vi "RIO control block_Dev_1.0.vi"() -> ()   [LabVIEW 2013]
uses:
  <vilib>/NI/Current Value Table/Type Defs/File Format.ctl
  <vilib>/NI/Current Value Table/Type Defs/Single Tag.ctl
  <vilib>/NI/Current Value Table/Type Defs/Data Types.ctl
  <vilib>/NI/Current Value Table/Type Defs/Tag Grouping set.ctl
  <vilib>/NI/Current Value Table/Type Defs/Group Data.ctl
  <vilib>/NI/Current Value Table/Read tags into grouped data.vi
  <vilib>/NI/Current Value Table/Write grouped data to tags.vi
  <vilib>/NI/Current Value Table/Read Index Set.vi
  <vilib>/NI/Current Value Table/DataTypes/Double_Read Index Set.vi
  <vilib>/NI/Current Value Table/DataTypes/Array of String_Read Index Set.vi
  <vilib>/NI/Current Value Table/DataTypes/Array of Boolean_Read Index Set.vi
  <vilib>/NI/Current Value Table/DataTypes/Array of Single_Read Index Set.vi
  <vilib>/NI/Current Value Table/DataTypes/Array of Double_Read Index Set.vi
  <vilib>/NI/Current Value Table/DataTypes/Array of I8_Read Index Set.vi
  <vilib>/NI/Current Value Table/DataTypes/Array of I16_Read Index Set.vi
  <vilib>/NI/Current Value Table/DataTypes/Array of I32_Read Index Set.vi
  <vilib>/NI/Current Value Table/DataTypes/Array of I64_Read Index Set.vi
  <vilib>/NI/Current Value Table/DataTypes/Array of U64_Read Index Set.vi
  <vilib>/NI/Current Value Table/DataTypes/Array of U32_Read Index Set.vi
  <vilib>/NI/Current Value Table/DataTypes/Array of U16_Read Index Set.vi
  <vilib>/NI/Current Value Table/DataTypes/Array of U8_Read Index Set.vi
  <vilib>/NI/Current Value Table/DataTypes/Boolean_Read Index Set.vi
  <vilib>/NI/Current Value Table/DataTypes/String_Read Index Set.vi
  <vilib>/NI/Current Value Table/DataTypes/U8_Read Index Set.vi
  <vilib>/NI/Current Value Table/DataTypes/U16_Read Index Set.vi
  <vilib>/NI/Current Value Table/DataTypes/U32_Read Index Set.vi
  <vilib>/NI/Current Value Table/DataTypes/U64_Read Index Set.vi
  <vilib>/NI/Current Value Table/DataTypes/I8_Read Index Set.vi
  <vilib>/NI/Current Value Table/DataTypes/I16_Read Index Set.vi
  <vilib>/NI/Current Value Table/DataTypes/I32_Read Index Set.vi
  <vilib>/NI/Current Value Table/DataTypes/I64_Read Index Set.vi
  <vilib>/NI/Current Value Table/DataTypes/Single_Read Index Set.vi
  <vilib>/NI/Current Value Table/Write Index Set.vi
  <vilib>/NI/Current Value Table/DataTypes/Double_Write Index Set.vi
  <vilib>/NI/Current Value Table/DataTypes/Array of String_Write Index Set.vi
  <vilib>/NI/Current Value Table/DataTypes/Array of Boolean_Write Index Set.vi
  <vilib>/NI/Current Value Table/DataTypes/Array of Single_Write Index Set.vi
  <vilib>/NI/Current Value Table/DataTypes/Array of Double_Write Index Set.vi
  <vilib>/NI/Current Value Table/DataTypes/Array of I8_Write Index Set.vi
  <vilib>/NI/Current Value Table/DataTypes/Array of I16_Write Index Set.vi
  <vilib>/NI/Current Value Table/DataTypes/Array of I32_Write Index Set.vi
  <vilib>/NI/Current Value Table/DataTypes/Array of I64_Write Index Set.vi
  <vilib>/NI/Current Value Table/DataTypes/Array of U64_Write Index Set.vi
  <vilib>/NI/Current Value Table/DataTypes/Array of U32_Write Index Set.vi
  <vilib>/NI/Current Value Table/DataTypes/Array of U16_Write Index Set.vi
  <vilib>/NI/Current Value Table/DataTypes/Array of U8_Write Index Set.vi
  <vilib>/NI/Current Value Table/DataTypes/Boolean_Write Index Set.vi
  <vilib>/NI/Current Value Table/DataTypes/String_Write Index Set.vi
  <vilib>/NI/Current Value Table/DataTypes/U8_Write Index Set.vi
  <vilib>/NI/Current Value Table/DataTypes/U16_Write Index Set.vi
  <vilib>/NI/Current Value Table/DataTypes/U32_Write Index Set.vi
  <vilib>/NI/Current Value Table/DataTypes/U64_Write Index Set.vi
  <vilib>/NI/Current Value Table/DataTypes/I8_Write Index Set.vi
  <vilib>/NI/Current Value Table/DataTypes/I16_Write Index Set.vi
  <vilib>/NI/Current Value Table/DataTypes/I32_Write Index Set.vi
  <vilib>/NI/Current Value Table/DataTypes/I64_Write Index Set.vi
  <vilib>/NI/Current Value Table/DataTypes/Single_Write Index Set.vi
  <vilib>/NI/Current Value Table/FGVs/Group Memory.vi
  <vilib>/NI/Current Value Table/Memory Block.vi
  <vilib>/NI/Current Value Table/DataTypes/Double_Memory Block.vi
  <vilib>/NI/Current Value Table/DataTypes/Array of String_Memory Block.vi
  <vilib>/NI/Current Value Table/DataTypes/Array of Boolean_Memory Block.vi
  <vilib>/NI/Current Value Table/DataTypes/Array of Single_Memory Block.vi
  <vilib>/NI/Current Value Table/DataTypes/Array of Double_Memory Block.vi
  <vilib>/NI/Current Value Table/DataTypes/Array of I8_Memory Block.vi
  <vilib>/NI/Current Value Table/DataTypes/Array of I16_Memory Block.vi
  <vilib>/NI/Current Value Table/DataTypes/Array of I32_Memory Block.vi
  <vilib>/NI/Current Value Table/DataTypes/Array of I64_Memory Block.vi
  <vilib>/NI/Current Value Table/DataTypes/Array of U64_Memory Block.vi
  <vilib>/NI/Current Value Table/DataTypes/Array of U32_Memory Block.vi
  <vilib>/NI/Current Value Table/DataTypes/Array of U16_Memory Block.vi
  <vilib>/NI/Current Value Table/DataTypes/Array of U8_Memory Block.vi
  <vilib>/NI/Current Value Table/DataTypes/Boolean_Memory Block.vi
  <vilib>/NI/Current Value Table/DataTypes/String_Memory Block.vi
  <vilib>/NI/Current Value Table/DataTypes/U8_Memory Block.vi
  <vilib>/NI/Current Value Table/DataTypes/U16_Memory Block.vi
  <vilib>/NI/Current Value Table/DataTypes/U32_Memory Block.vi
  <vilib>/NI/Current Value Table/DataTypes/U64_Memory Block.vi
  <vilib>/NI/Current Value Table/DataTypes/I8_Memory Block.vi
  <vilib>/NI/Current Value Table/DataTypes/I16_Memory Block.vi
  <vilib>/NI/Current Value Table/DataTypes/I32_Memory Block.vi
  <vilib>/NI/Current Value Table/DataTypes/I64_Memory Block.vi
  <vilib>/NI/Current Value Table/DataTypes/Single_Memory Block.vi
  <vilib>/NI/Current Value Table/Current Value Table.lvlib
  <vilib>/ptbypt/NI_PtbyPt.lvlib
panel:
  out "HH Alarms":bool[](array[boolean])
  out "Double":dbl[](array[numeric])
  out "CVT Tags":T1
  out "Boolean 5":bool
  out "Boolean 4":bool
  out "Boolean 2":bool
  in  "stop 3":bool
  out "mean 2":dbl format="%0.2f"
  in  "stop 2":bool
  in  "Boolean":bool
  in  "Numeric 7":dbl
  in  "Numeric 6":dbl
  in  "Numeric 4":dbl
  in  "Numeric 3":dbl
  in  "Numeric 2":dbl
  in  "Numeric":dbl
  out "mean":dbl format="%0.2f"
  in  "stop":bool
  # "HH"
  # "HH"
  # "HH"
  # "HH"
  # "TI-101"
  # "PI-101"
  # "PI-102"
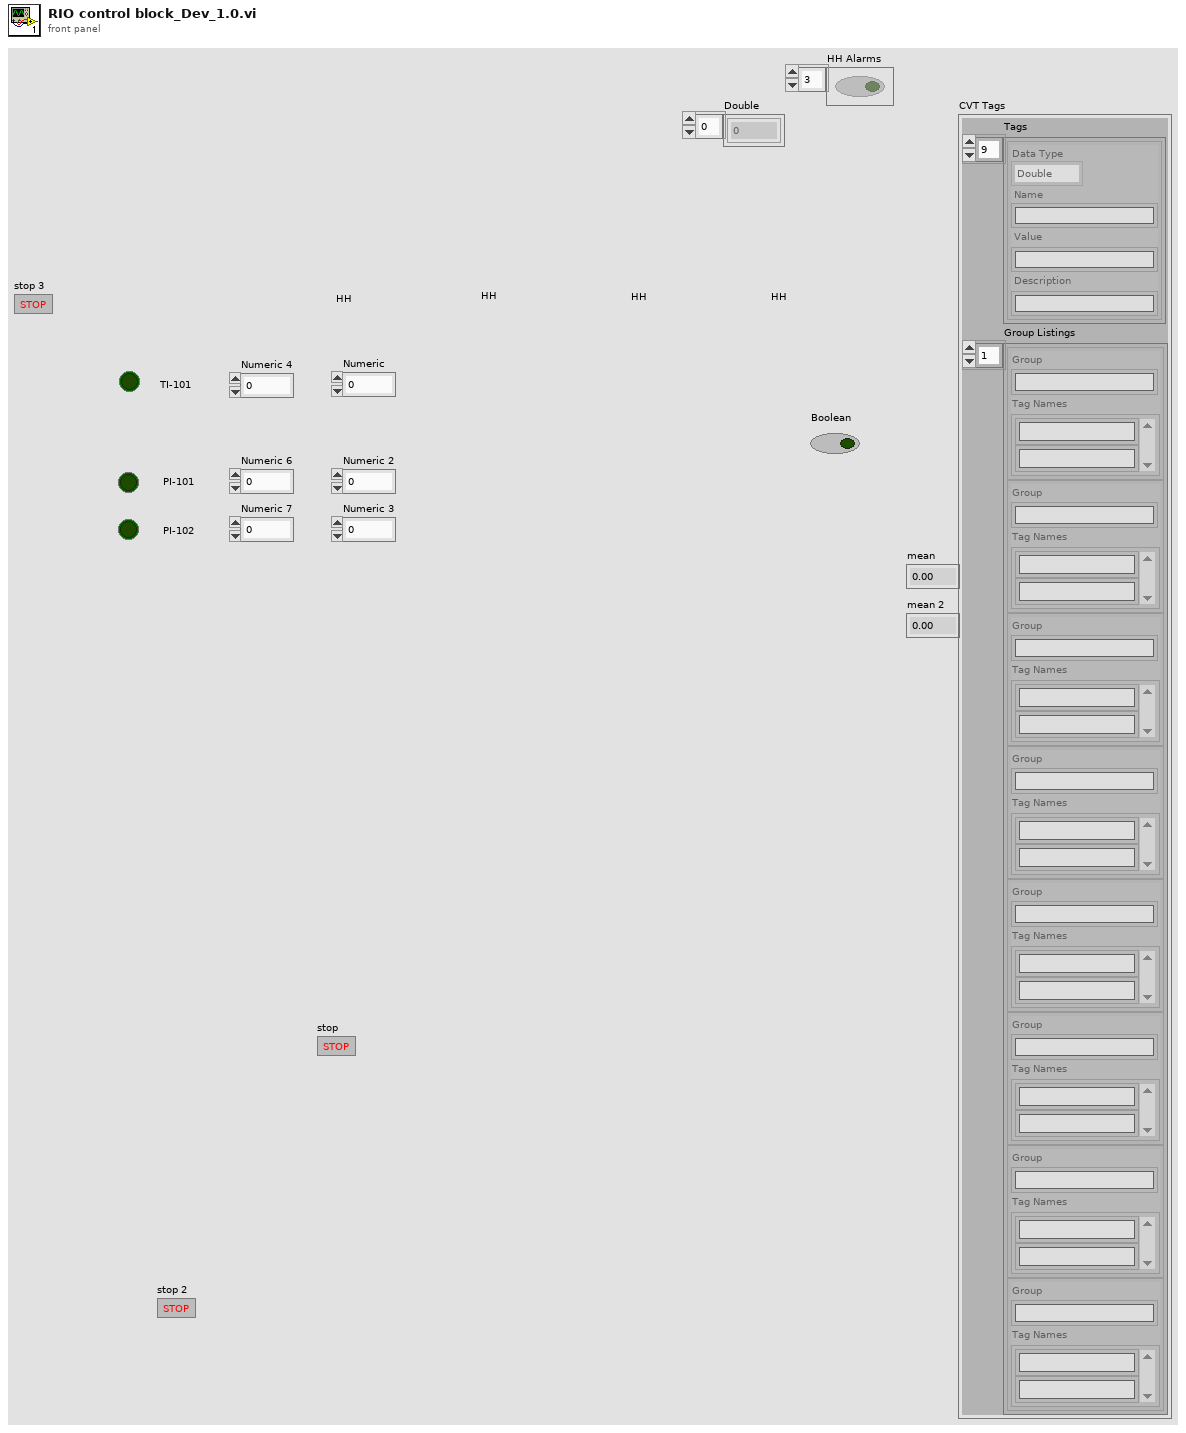
[diagram p1: front panel]
types:
  T1 = typedef "Current Value Table.lvlib/File Format.ctl" = cluster{"Tags":T2[], "Group Listings":T4[]}
  T2 = typedef "Current Value Table.lvlib/Single Tag.ctl" = cluster{"Data Type":T3, "Name":string, "Value":string, "Description":string}
  T3 = typedef "Current Value Table.lvlib/Data Types.ctl" = enum16{"Double", "Single", "I64", "I32", "I16", "I8", "U64", "U32", "U16", "U8", "String", "Boolean", "Array of U8", "Array of U16", "Array of U32", "Array of U64", "Array of I64", "Array of I32", "Array of I16", "Array of I8", "Array of Double", "Array of Single", "Array of Boolean", "Array of String"}
  T4 = typedef "Current Value Table.lvlib/Tag Grouping set.ctl" = cluster{"Group":string, "Tag Names":string[]}
  T5 = typedef "Current Value Table.lvlib/Group Data.ctl" = cluster{"Double":dbl[], "Single":sgl[], "I64":i64[], "I32":i32[], "I16":i16[], "I8":i8[], "U64":u64[], "U32":u32[], "U16":u16[], "U8":u8[], "String":string[], "Boolean":bool[], "Array of U8":cluster{"U8 Array":u8[]}[], "Array of U16":cluster{"U16 Array":u16[]}[], "Array of U32":cluster{"U32 Array":u32[]}[], "Array of U64":cluster{"U64 Array":u64[]}[], "Array of I64":cluster{"I64 Array":i64[]}[], "Array of I32":cluster{"I32 Array":i32[]}[], "Array of I16":cluster{"I16 Array":i16[]}[], "Array of I8":cluster{"I8 Array":i8[]}[], "Array of Double":cluster{"DBL Array":dbl[]}[], "Array of Single":cluster{"SGL Array":sgl[]}[], "Array of Boolean":cluster{"Boolean Array":bool[]}[], "Array of String":cluster{"String Array":string[]}[]}
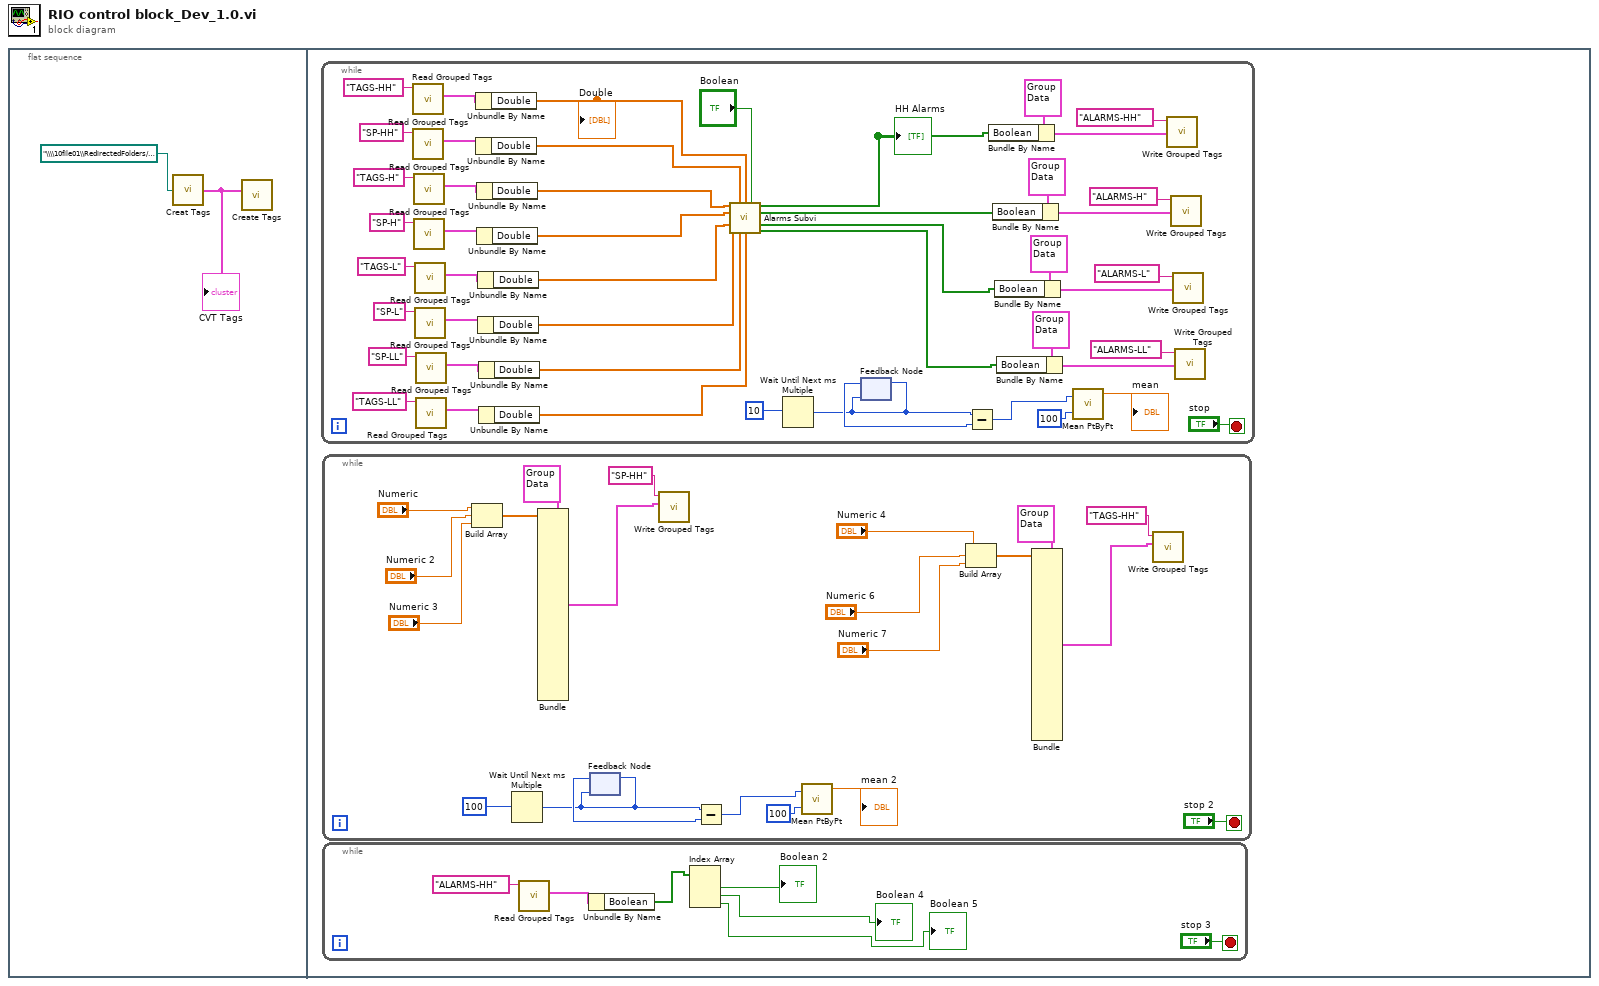
[diagram p0: block diagram]
diagram:
  n1 = flat-sequence {
    frame #0 {
      n2 = call "Creat Tags.vi"("File Path"=path "\\\\10file01\\RedirectedFolders/mike.delaplain/Documents/LabVIEW/SDF Small Gasifier/Tags_Dev.csv" ("file path (dialog if empty)")) -> ("CVT Tags"=w1:T1)
      "CVT Tags" <- w1
      n3 = call <vilib>:"Create Tags.vi"("CVT Tags to Create"=w1) -> ()  [unwired: 10 in, 1 out]
    }
    frame #1 {
      n4 = while {
        stop <- "stop" stop-if-true
        n5 = call <vilib>:"Read Grouped Tags.vi"("Group"="TAGS-HH") -> ("Data"=w75:T5)  [unwired: 9 in, 1 out]
        n6 = call <vilib>:"Read Grouped Tags.vi"("Group"="SP-HH") -> ("Data"=w74:T5)  [unwired: 9 in, 1 out]
        n7 = call <vilib>:"Read Grouped Tags.vi"("Group"="TAGS-H") -> ("Data"=w62:T5)  [unwired: 9 in, 1 out]
        n8 = call <vilib>:"Read Grouped Tags.vi"("Group"="SP-H") -> ("Data"=w61:T5)  [unwired: 9 in, 1 out]
        n9 = call <vilib>:"Read Grouped Tags.vi"("Group"="TAGS-L") -> ("Data"=w58:T5)  [unwired: 9 in, 1 out]
        n10 = call <vilib>:"Read Grouped Tags.vi"("Group"="SP-L") -> ("Data"=w57:T5)  [unwired: 9 in, 1 out]
        n11 = call <vilib>:"Read Grouped Tags.vi"("Group"="SP-LL") -> ("Data"=w54:T5)  [unwired: 9 in, 1 out]
        n12 = call <vilib>:"Read Grouped Tags.vi"("Group"="TAGS-LL") -> ("Data"=w53:T5)  [unwired: 9 in, 1 out]
        n13 = Unbundle By Name(w75) -> ("Double"=w52:dbl[])
        "Double" <- w52
        n14 = Unbundle By Name(w74) -> ("Double"=w51:dbl[])
        n15 = Unbundle By Name(w62) -> ("Double"=w50:dbl[])
        n16 = Unbundle By Name(w61) -> ("Double"=w49:dbl[])
        n17 = Unbundle By Name(w58) -> ("Double"=w48:dbl[])
        n18 = Unbundle By Name(w57) -> ("Double"=w47:dbl[])
        n19 = Unbundle By Name(w54) -> ("Double"=w46:dbl[])
        n20 = Unbundle By Name(w53) -> ("Double"=w45:dbl[])
        n21 = call "Alarms Subvi.vi"("H Tags"=w50, "HH SP"=w51, "HH Tags"=w52, "Reset"="Boolean", "H SP"=w49, "LTags"=w48, "L SP"=w47, "LL SP"=w46, "LL Tage"=w45) -> ("HH Alarms"=w35:bool[], "H Alarms"=w34:bool[], "L Alarms"=w33:bool[], "LL Alarms"=w32:bool[])  [unwired: 3 in]
        "HH Alarms" <- w35
        n22 = Wait Until Next ms Multiple(millisecond multiple=u32 10 ("millisecond timer value")) -> (millisecond timer value=w68:u32)
        n23 = feedback #1(w68) -> (w70:u32)
        n24 = feedback-in #1(w68) -> ()
        n25 = Subtract(x=w68, y=w70) -> (x-y=w69:u32)
        n26 = Bundle By Name(cluster=T5 {"Double"=[], "Single"=[], "I64"=[], "I32"=[], "I16"=[], "I8"=[], "U64"=[], "U32"=[], "U16"=[], "U8"=[], "String"=[], "Boolean"=[], "Array of U8"=[], "Array of U16"=[], "Array of U32"=[], "Array of U64"=[], "Array of I64"=[], "Array of I32"=[], "Array of I16"=[], "Array of I8"=[], "Array of Double"=[], "Array of Single"=[], "Array of Boolean"=[], "Array of String"=[]} ("Data"), "Boolean"=w35) -> (w42:T5)
        n27 = Bundle By Name(cluster=T5 {"Double"=[], "Single"=[], "I64"=[], "I32"=[], "I16"=[], "I8"=[], "U64"=[], "U32"=[], "U16"=[], "U8"=[], "String"=[], "Boolean"=[], "Array of U8"=[], "Array of U16"=[], "Array of U32"=[], "Array of U64"=[], "Array of I64"=[], "Array of I32"=[], "Array of I16"=[], "Array of I8"=[], "Array of Double"=[], "Array of Single"=[], "Array of Boolean"=[], "Array of String"=[]} ("Data"), "Boolean"=w34) -> (w65:T5)
        n28 = Bundle By Name(cluster=T5 {"Double"=[], "Single"=[], "I64"=[], "I32"=[], "I16"=[], "I8"=[], "U64"=[], "U32"=[], "U16"=[], "U8"=[], "String"=[], "Boolean"=[], "Array of U8"=[], "Array of U16"=[], "Array of U32"=[], "Array of U64"=[], "Array of I64"=[], "Array of I32"=[], "Array of I16"=[], "Array of I8"=[], "Array of Double"=[], "Array of Single"=[], "Array of Boolean"=[], "Array of String"=[]} ("Data"), "Boolean"=w33) -> (w39:T5)
        n29 = Bundle By Name(cluster=T5 {"Double"=[], "Single"=[], "I64"=[], "I32"=[], "I16"=[], "I8"=[], "U64"=[], "U32"=[], "U16"=[], "U8"=[], "String"=[], "Boolean"=[], "Array of U8"=[], "Array of U16"=[], "Array of U32"=[], "Array of U64"=[], "Array of I64"=[], "Array of I32"=[], "Array of I16"=[], "Array of I8"=[], "Array of Double"=[], "Array of Single"=[], "Array of Boolean"=[], "Array of String"=[]} ("Data"), "Boolean"=w32) -> (w36:T5)
        n30 = call <vilib>:"Mean PtByPt.vi"("x"=w69, "sample length"=100) -> ("mean"=→"mean":dbl)  [unwired: 2 in, 1 out]
        n31 = call <vilib>:"Write Grouped Tags.vi"("Data"=w42, "Group"="ALARMS-HH") -> ()  [unwired: 9 in, 1 out]
        n32 = call <vilib>:"Write Grouped Tags.vi"("Data"=w65, "Group"="ALARMS-H") -> ()  [unwired: 9 in, 1 out]
        n33 = call <vilib>:"Write Grouped Tags.vi"("Data"=w39, "Group"="ALARMS-L") -> ()  [unwired: 9 in, 1 out]
        n34 = call <vilib>:"Write Grouped Tags.vi"("Data"=w36, "Group"="ALARMS-LL") -> ()  [unwired: 9 in, 1 out]
      }
      n35 = while {
        stop <- "stop 2" stop-if-true
        n36 = Build Array("Numeric", "Numeric 2", "Numeric 3") -> (w25:dbl[])
        n37 = Wait Until Next ms Multiple(millisecond multiple=u32 100 ("millisecond timer value")) -> (millisecond timer value=w18:u32)
        n38 = Bundle(cluster=T5 {"Double"=[], "Single"=[], "I64"=[], "I32"=[], "I16"=[], "I8"=[], "U64"=[], "U32"=[], "U16"=[], "U8"=[], "String"=[], "Boolean"=[], "Array of U8"=[], "Array of U16"=[], "Array of U32"=[], "Array of U64"=[], "Array of I64"=[], "Array of I32"=[], "Array of I16"=[], "Array of I8"=[], "Array of Double"=[], "Array of Single"=[], "Array of Boolean"=[], "Array of String"=[]} ("Data"), "Double"=w25) -> (w24:T5)  [unwired: 23 in]
        n39 = feedback #2(w18) -> (w20:u32)
        n40 = feedback-in #2(w18) -> ()
        n41 = call <vilib>:"Write Grouped Tags.vi"("Data"=w24, "Group"="SP-HH") -> ()  [unwired: 9 in, 1 out]
        n42 = Subtract(x=w18, y=w20) -> (x-y=w19:u32)
        n43 = call <vilib>:"Mean PtByPt.vi"("x"=w19, "sample length"=100) -> ("mean"=→"mean 2":dbl)  [unwired: 2 in, 1 out]
        n44 = Build Array("Numeric 4", "Numeric 6", "Numeric 7") -> (w14:dbl[])
        n45 = Bundle(cluster=T5 {"Double"=[], "Single"=[], "I64"=[], "I32"=[], "I16"=[], "I8"=[], "U64"=[], "U32"=[], "U16"=[], "U8"=[], "String"=[], "Boolean"=[], "Array of U8"=[], "Array of U16"=[], "Array of U32"=[], "Array of U64"=[], "Array of I64"=[], "Array of I32"=[], "Array of I16"=[], "Array of I8"=[], "Array of Double"=[], "Array of Single"=[], "Array of Boolean"=[], "Array of String"=[]} ("Data"), "Double"=w14) -> (w13:T5)  [unwired: 23 in]
        n46 = call <vilib>:"Write Grouped Tags.vi"("Data"=w13, "Group"="TAGS-HH") -> ()  [unwired: 9 in, 1 out]
      }
      n47 = while {
        stop <- "stop 3" stop-if-true
        n48 = call <vilib>:"Read Grouped Tags.vi"("Group"="ALARMS-HH") -> ("Data"=w7:T5)  [unwired: 9 in, 1 out]
        n49 = Unbundle By Name(w7) -> ("Boolean"=w6:bool[])
        n50 = Index Array(array=w6) -> (element #1=→"Boolean 2":bool, element #2=→"Boolean 4":bool, element #3=→"Boolean 5":bool)  [unwired: 3 in]
      }
    }
  }
